vi "BuildSendQueryString.vi"(10 "sendMessage":T1, 11 "Token":string) -> (3 "QueryStringOut":string)   [LabVIEW 2019]
uses:
  TypeDefs/sendMessage.ctl
  TypeDefs/Method.ctl
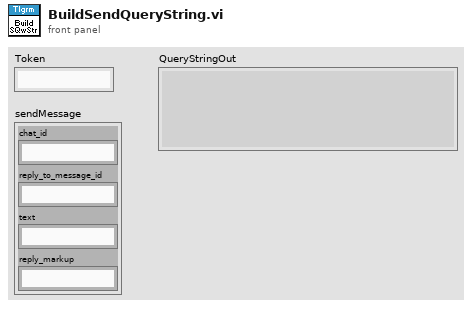
[diagram p1: front panel]
types:
  T1 = typedef "sendMessage.ctl" = cluster{"chat_id":string, "reply_to_message_id":string, "text":string, "reply_markup":string}
  T2 = typedef "Method.ctl" = string
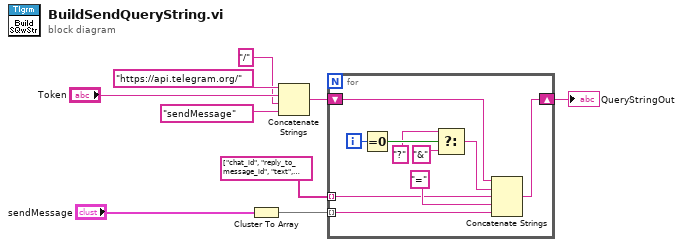
[diagram p0: block diagram]
diagram:
  n1 = Cluster To Array(cluster="sendMessage") -> (array=w4:string[])
  n2 = Concatenate Strings("https://api.telegram.org/" ("URL"), "Token", "/" ("URL"), T2 "sendMessage" ("Method")) -> (w6:string)
  n3 = for {
    shift-right: [w13] -> w9
    shift-left: w6 -> [w12]
    tunnel: w4 -> [w11] mode=indexing
    tunnel: string[] ["chat_id", "reply_to_message_id", "text", "reply_markup"] ("sendMessageParam") -> [w10] mode=indexing
    i -> [w15]
    n4 = Equal To 0?(x=w15) -> (x = 0?=w18:bool)
    n5 = Select(t="?", s=w18, f="&") -> (s? t:f=w14:string)
    n6 = Concatenate Strings(w12, w14, w10, "=" ("string"), w11) -> (w13:string)
  }
  "QueryStringOut" <- w9
